vi "TwoBallAutoMain.vi"   [LabVIEW 2015]
uses:
  <vilib>/Rock Robotics/WPI/DriverStation/WPI_DriverStationRobotMode2.ctl
  Utilities/MotorPositionGlobals.vi
  Utilities/AutoVars.vi
  TwoBallAutoGlobals.vi
  Utilities/VisionGlobals.vi
  navx-mxp/labview/navX Library v2/navX Library v2.lvlib
types:
  T1 = enum16{"WaitForInput", "StartIntake", "LowerArm", "IntakeBall", "TurnAndZeroEnc", "DriveForward", "RecordGyro", "TargetAndLoad", "Shoot", "TurnBack", "BackUpAndIntake", "IntakeBall2", "DriveForward2", "TargetAndLoad2", "Shoot2", "End"}
  T2 = typedef "WPI_DriverStationRobotMode2.ctl" = enum16{"Autonomous Disabled", "Autonomous Enabled", "Teleop Disabled", "Teleop Enabled", "Disconnected", "Finish", "Test Disabled", "Test Enabled", "Emergency Stopped"}
  T3 = typedef "WPI_MotorControlDeviceRef.ctl" = cluster{"DeviceStatus":errorcluster, "Type":T4, "PWM":cluster{"PWM Channel":T5, "DeadBand":T6}, "CAN":cluster{"Device Number":u8, "Control Mode":T7, "Semaphore":T8, "Max Vout":dbl, "TalonSRX Control Mode":T9}, "Invert":bool}
  T4 = typedef "WPI_MotorControlType.ctl" = enum16{"PWM", "CAN", "CANTalonSRX"}
  T5 = typedef "FPGA_DIOPWMChannel.ctl" = enum8{"PWM 0", "PWM 1", "PWM 2", "PWM 3", "PWM 4", "PWM 5", "PWM 6", "PWM 7", "PWM 8", "PWM 9", "PWM MXP 0", "PWM MXP 1", "PWM MXP 2", "PWM MXP 3", "PWM MXP 4", "PWM MXP 5", "PWM MXP 6", "PWM MXP 7", "PWM MXP 8", "PWM MXP 9", "Invalid"}
  T6 = typedef "WPI_PWMDeadband.ctl" = cluster{"Name":string, "maxPositivePwm":i32, "minPositivePwm":i32, "centerPwm":i32, "maxNegativePwm":i32, "minNegativePwm":i32, "angularRange":u16}
  T7 = typedef "WPI_CANJaguar_ControlMode.ctl" = enum8{"Percent VBus", "Current", "Speed", "Position", "Voltage"}
  T8 = typedef "Semaphore RefNum" = refnum<k1>
  T9 = typedef "WPI_CANTalonSRX_APIControlMode.ctl" = enum8{"Percent VBus", "Speed", "Position", "Slave", "Unchanged / Invalid", "Voltage Compensation", "Current", "Motion Profile"}
  T10 = typedef "navX Library v2.lvlib/Z900_navX_DeviceTypeDef.ctl" = cluster{"Interface":cluster{"Protocol":T11, "Update Rate (4Hz-100Hz)":u8, "navX Open TypeDef":variant}, "Notify Packet":refnum<notifier>, "Loop VI Refnum":refnum<vi>, "Ready to Close Occurrence Refnum":refnum<k4>}
  T11 = typedef "navX Library v2.lvlib/Z900_navX_ProtocolTypeDef.ctl" = enum16{"SERIAL", "I2C", "SPI"}
  T12 = cluster{"Yaw":dbl, "Roll":dbl, "Pitch":dbl, "Heading":dbl, "Fused Heading":dbl}
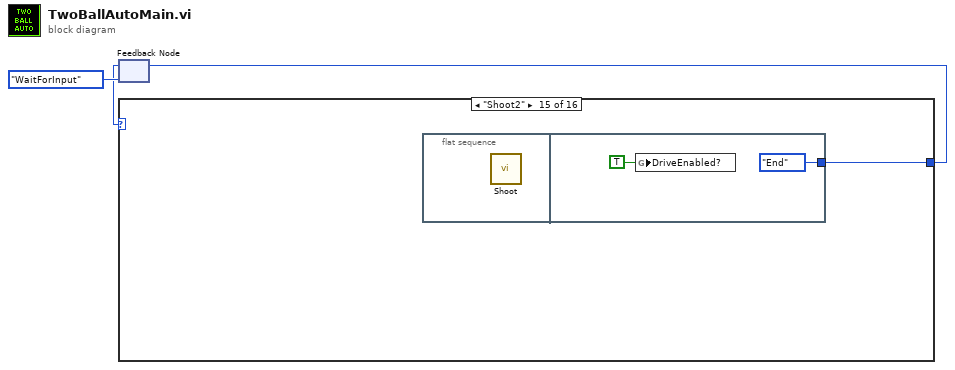
[diagram p0: block diagram]
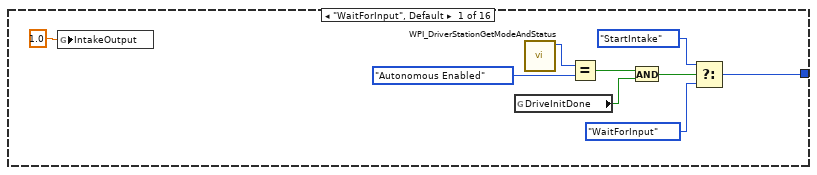
[diagram p2: hidden frame]
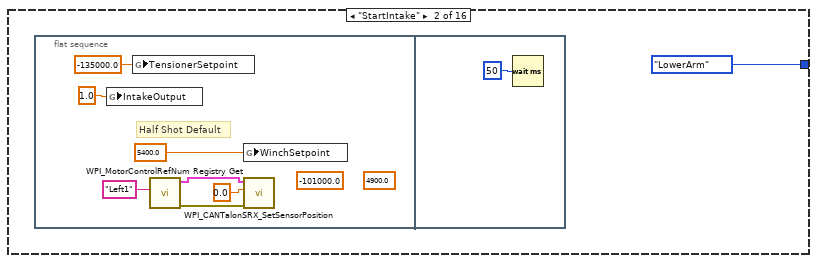
[diagram p3: hidden frame]
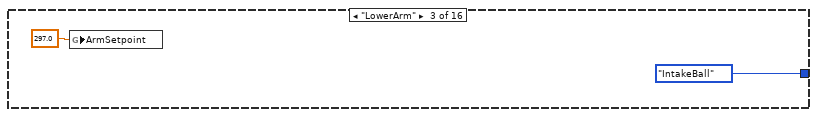
[diagram p4: hidden frame]
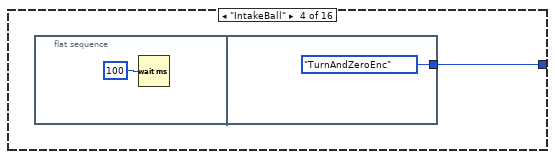
[diagram p5: hidden frame]
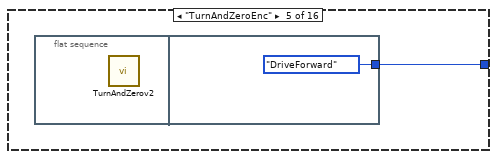
[diagram p6: hidden frame]
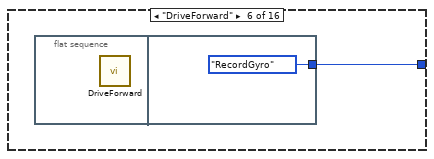
[diagram p7: hidden frame]
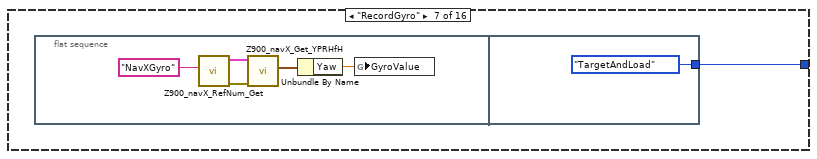
[diagram p8: hidden frame]
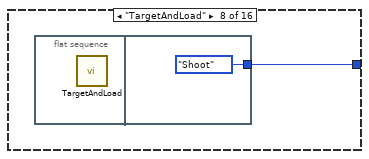
[diagram p9: hidden frame]
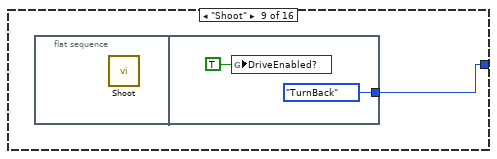
[diagram p10: hidden frame]
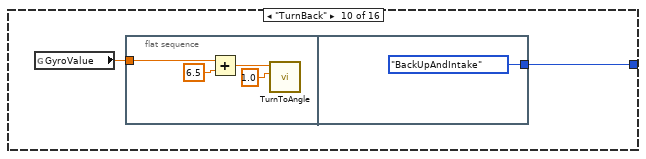
[diagram p11: hidden frame]
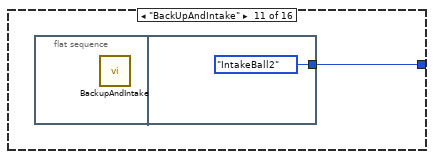
[diagram p12: hidden frame]
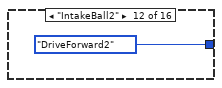
[diagram p13: hidden frame]
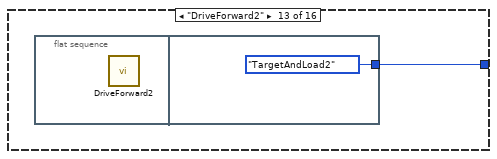
[diagram p14: hidden frame]
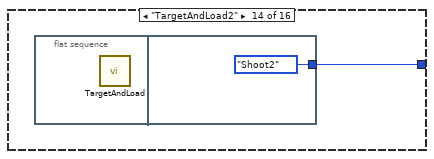
[diagram p15: hidden frame]
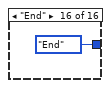
[diagram p16: hidden frame]
diagram:
  n1 = feedback #1(T1."WaitForInput" ("Enum")) -> (w1:T1)
  n2 = case shown="\"Shoot2\"" w1 {
    tunnel: [w5 T1."LowerArm" ("Enum") T1."IntakeBall" ("Enum") w24 w27 w29 w31 w38 w40 w43 w50 T1."DriveForward2" ("Enum") w53 w55 w57 T1."End" ("Enum")] -> w3
    frame "WaitForInput", Default {
      n3 = global write "MotorPositionGlobals.vi" "IntakeOutput"(1.0 ("IntakeOutput")) -> ()
      n4 = global read "AutoVars.vi" "DriveInitDone"() -> (w9:bool)
      n5 = call <vilib>:"WPI_DriverStationGetModeAndStatus.vi"() -> ("Robot Mode"=w12:T2)  [unwired: 10 in, 1 out]
      n6 = Equal?(x=w12, y=WPI_DriverStationRobotMode2."Autonomous Enabled" ("Robot Mode")) -> (x = y?=w10:bool)
      n7 = And(x=w10, y=w9) -> (x .and. y?=w8:bool)
      n8 = Select(t=T1."StartIntake" ("Enum"), s=w8, f=T1."WaitForInput" ("Enum")) -> (s? t:f=w5:T1)
    }
    frame "StartIntake" {
      n9 = flat-sequence {
        frame #0 {
          (unwired) 4900.0 ("WinchPosition")
          (unwired) -101000.0 ("TensionerSetpoint")
          # "Half Shot Default"
          n10 = global write "MotorPositionGlobals.vi" "IntakeOutput"(1.0 ("IntakeOutput")) -> ()
          n11 = global write "MotorPositionGlobals.vi" "TensionerSetpoint"(-135000.0 ("TensionerSetpoint")) -> ()
          n12 = call <vilib>:"WPI_MotorControlRefNum Registry Get.vi"("refnum name"="Left1") -> ("error out"=w15:errorcluster, "MotorControlDevRef"=w16:T3)  [unwired: 9 in]
          n13 = global write "MotorPositionGlobals.vi" "WinchSetpoint"(5400.0 ("WinchPosition")) -> ()
          n14 = call <vilib>:"WPI_CANTalonSRX_SetSensorPosition.vi"("error in (no error)"=w15, "New Sensor Position"=0.0, "CAN Talon SRX Ref"=w16) -> ()  [unwired: 7 in, 2 out]
        }
        frame #1 {
          n15 = Wait (ms)(milliseconds to wait=u32 50) -> ()  [unwired: 1 out]
        }
      }
    }
    frame "LowerArm" {
      n16 = global write "MotorPositionGlobals.vi" "ArmSetpoint"(297.0 ("ArmSetpoint")) -> ()
    }
    frame "IntakeBall" {
      n17 = flat-sequence {
        tunnel: [T1."TurnAndZeroEnc" ("Enum")] -> w24
        frame #0 {
          n18 = Wait (ms)(milliseconds to wait=u32 100) -> ()  [unwired: 1 out]
        }
        frame #1 {
        }
      }
    }
    frame "TurnAndZeroEnc" {
      n19 = flat-sequence {
        tunnel: [T1."DriveForward" ("Enum")] -> w27
        frame #0 {
          n20 = call "TurnAndZerov2.vi"() -> ()  [unwired: 12 in]
        }
        frame #1 {
        }
      }
    }
    frame "DriveForward" {
      n21 = flat-sequence {
        tunnel: [T1."RecordGyro" ("Enum")] -> w29
        frame #0 {
          n22 = call "DriveForward.vi"() -> ()  [unwired: 12 in]
        }
        frame #1 {
        }
      }
    }
    frame "RecordGyro" {
      n23 = flat-sequence {
        tunnel: [T1."TargetAndLoad" ("Enum")] -> w31
        frame #0 {
          n24 = call "Z900_navX_RefNum_Get.vi"("refnum name"="NavXGyro") -> ("error out"=w35:errorcluster, "navX Device"=w36:T10)  [unwired: 9 in]
          n25 = call "Z900_navX_Get_YPRHfH.vi"("error in (no error)"=w35, "navX Device"=w36) -> ("YRPHfH"=w33:T12)  [unwired: 6 in, 3 out]
          n26 = Unbundle By Name(w33) -> ("Yaw"=w32:dbl)
          n27 = global write "TwoBallAutoGlobals.vi" "GyroValue"(w32) -> ()
        }
        frame #1 {
        }
      }
    }
    frame "TargetAndLoad" {
      n28 = flat-sequence {
        tunnel: [T1."Shoot" ("Enum")] -> w38
        frame #0 {
          n29 = call "TargetAndLoad.vi"() -> ()  [unwired: 1 in]
        }
        frame #1 {
        }
      }
    }
    frame "Shoot" {
      n30 = flat-sequence {
        tunnel: [T1."TurnBack" ("Enum")] -> w40
        frame #0 {
          n31 = call "Shoot.vi"() -> ()  [unwired: 12 in]
        }
        frame #1 {
          n32 = global write "VisionGlobals.vi" "DriveEnabled?"(TRUE ("DriveEnabled?")) -> ()
        }
      }
    }
    frame "TurnBack" {
      n33 = global read "TwoBallAutoGlobals.vi" "GyroValue"() -> (w44:dbl)
      n34 = flat-sequence {
        tunnel: w44 -> [w47]
        tunnel: [T1."BackUpAndIntake" ("Enum")] -> w43
        frame #0 {
          n35 = Add(x=w47, y=6.5) -> (x+y=w46:dbl)
          n36 = call "TurnToAngle.vi"("AllowedDeviation"=1.0, "GyroValue"=w46) -> ()  [unwired: 10 in]
        }
        frame #1 {
        }
      }
    }
    frame "BackUpAndIntake" {
      n37 = flat-sequence {
        tunnel: [T1."IntakeBall2" ("Enum")] -> w50
        frame #0 {
          n38 = call "BackupAndIntake.vi"() -> ()  [unwired: 2 in]
        }
        frame #1 {
        }
      }
    }
    frame "IntakeBall2" {
    }
    frame "DriveForward2" {
      n39 = flat-sequence {
        tunnel: [T1."TargetAndLoad2" ("Enum")] -> w53
        frame #0 {
          n40 = call "DriveForward2.vi"() -> ()  [unwired: 2 in]
        }
        frame #1 {
        }
      }
    }
    frame "TargetAndLoad2" {
      n41 = flat-sequence {
        tunnel: [T1."Shoot2" ("Enum")] -> w55
        frame #0 {
          n42 = call "TargetAndLoad.vi"() -> ()  [unwired: 1 in]
        }
        frame #1 {
        }
      }
    }
    frame "Shoot2" {
      n43 = flat-sequence {
        tunnel: [T1."End" ("Enum")] -> w57
        frame #0 {
          n44 = call "Shoot.vi"() -> ()  [unwired: 12 in]
        }
        frame #1 {
          n45 = global write "VisionGlobals.vi" "DriveEnabled?"(TRUE ("DriveEnabled?")) -> ()
        }
      }
    }
    frame "End" {
    }
  }
  n46 = feedback-in #1(w3) -> ()
